vi "Init.vi"(8 "error in (no error)":errorcluster, 10 "VISA name":refnum<visa-resource-name>="GPIB::5::INSTR", 11 "VISA in":refnum<class "VISA.lvclass">) -> (0 "error out":errorcluster, 3 "VISA out":refnum<class "VISA.lvclass">)   [LabVIEW 2020, in "Low Level PSU With Tests.lvlib" / "VISA.lvclass"]
uses:
  VISA.lvclass
  VISA.lvclass/VISA.ctl
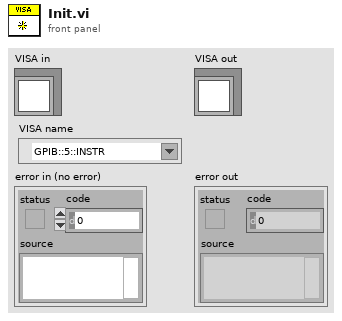
[diagram p1: front panel]
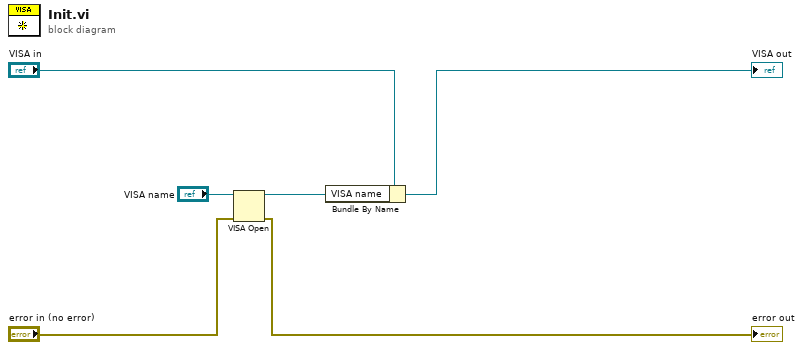
[diagram p0: block diagram]
diagram:
  n1 = VISA Open(error in (no error)="error in (no error)", VISA resource name="VISA name") -> (VISA resource name=w5:refnum<visa-resource-name>, error out=→"error out":errorcluster)  [unwired: 3 in]
  n2 = Bundle By Name(cluster="VISA in", "VISA name"=w5) -> (→"VISA out":refnum<class "VISA.lvclass">)
